vi "fill ring control with options.vi"(8 "error in (no error)":errorcluster, 10 "ring options":T1, 11 "Ring Ref":refnum<vi>[](array[refnum])) -> (0 "error out":errorcluster)   [LabVIEW 2024]
uses:
  config data.ctl
  API Config Files Management.lvlib
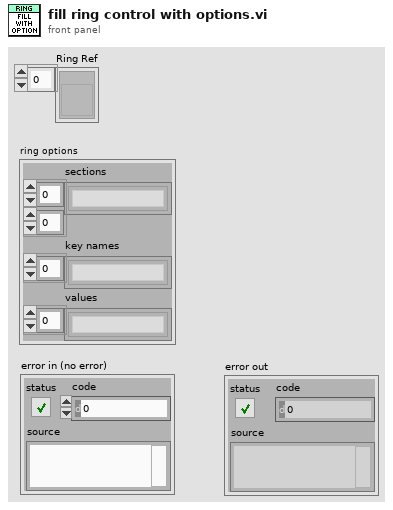
[diagram p1: front panel]
types:
  T1 = typedef "API Config Files Management.lvlib/config data.ctl" = cluster{"sections":string[][], "key names":string[], "values":string[]}
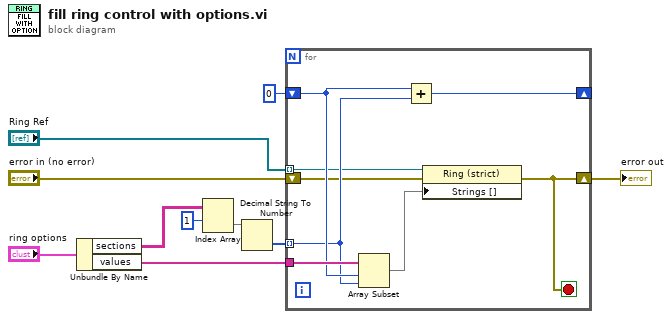
[diagram p0: block diagram]
diagram:
  n1 = Unbundle By Name("ring options") -> ("sections"=w5:string[][], "values"=w1:string[])
  n2 = Index Array(array=w5, index (row)=1) -> (element=w7:string[])  [unwired: 1 in]
  n3 = Decimal String To Number(string=w7) -> (number=w8:i32[])  [unwired: 2 in, 1 out]
  n4 = for {
    tunnel: w8 -> [w15] mode=indexing
    shift-right: [w18] -> _
    shift-left: 0 -> [w16]
    tunnel: w1 -> [w17]
    tunnel: "Ring Ref" -> [w14] mode=indexing
    shift-right: [w12] -> w10
    shift-left: "error in (no error)" -> [w11]
    stop <- w12 stop-if-true
    n5 = Array Subset(array=w17, index=w16, length=w15) -> (w13:string[])
    n6 = Add(x=w16, y=w15) -> (x+y=w18:i32)
    n7 = property on="Property Node" class="Ring (strict)"(reference=w14, error in=w11, "Strings []"=w13) -> (error out=w12:errorcluster)  [unwired: 1 out]
  }
  "error out" <- w10
